vi "check controller rectangle cases.vi"() -> ()   [LabVIEW 2017]
uses:
  <vilib>/Simulation/Scripting/Companion Diagram/SimConfigNode/SimParams.ctl
  <vilib>/Simulation/Scripting/Companion Diagram/SimConfigNode/_simSolvers.ctl
  <vilib>/Simulation/Implementation/Shared/SIMSCR Execution Mode.ctl
  <vilib>/Simulation/Param Hierarchy/Typedefs/SIMPH Param Control Actions.ctl
  <vilib>/Simulation/Implementation/Shared/NILVSim_ParamChanged.vi
  <vilib>/Simulation/Implementation/Shared/NILVSIM_BeginStep.vi
  <vilib>/Simulation/Implementation/Shared/NILVSim_Manager.vi
  <vilib>/Utility/error.llb/Clear Errors.vi
  <vilib>/Simulation/Implementation/Shared/NILVSim_FinalizeModel.vi
  <vilib>/DAQmx/read.llb/DAQmx Read (Counter DBL 1Chan 1Samp).vi
  <vilib>/DAQmx/read.llb/DAQmx Read (Digital Bool 1Line 1Point).vi
  917b7e52-755f-4d44-bea8-9e7c9beac24e.vi
  a58f9967-76f1-4ebc-ad3d-26e75a3ca160.vi
  <vilib>/DAQmx/write.llb/DAQmx Write (Analog DBL 1Chan 1Samp).vi
  <vilib>/DAQmx/create/channels.llb/DAQmx Create Channel (AO-Voltage-Basic).vi
  <vilib>/DAQmx/create/channels.llb/DAQmx Create Channel (DI-Digital Input).vi
  <vilib>/DAQmx/create/channels.llb/DAQmx Create Channel (CI-Count Edges).vi
  <vilib>/Simulation/Implementation/Shared/SIM Unbundle Sim Info.vi
  <vilib>/Simulation/Implementation/Shared/NILVSim_Initialize.vi
  <vilib>/Simulation/Utility/Implementation/NILVSim Get Time and IsAcceptedStep.vi
  <vilib>/Simulation/Implementation/Shared/SIMSH Read Queue.vi
  <vilib>/Simulation/Implementation/Shared/NILVSim_GetModelError.vi
  <vilib>/Simulation/Implementation/Shared/SIM Bundle Sim Info.vi
  <vilib>/DAQmx/miscellaneous.llb/DAQmx Fill In Error Info.vi
  <vilib>/Simulation/Implementation/XNodeFramework/SimXNode/SimX.xnode
  <vilib>/Simulation/Model Libraries/PID/SIM PID (Parallel).vi
  <vilib>/Simulation/Model Libraries/PID/SIM PID.vi
  <vilib>/Simulation/Scripting/Companion Diagram/SimConfigNode/SimDog.xnode
  <vilib>/Simulation/Model Libraries/PID/SIM PID (Academic).vi
  <vilib>/Simulation/Implementation/Shared/NI_SIM_Implementation.lvlib
panel:
  out "Boolean 3":bool
  out "temp height":dbl
  out "Boolean 2":bool
  out "reset":bool
  in  "checking re":bool
  in  "checking enums":T1(ring)
  in  "rectangle":bool
  in  "Boolean":bool
  out "prev index":dbl
  out "Point rectangle is drawing":dbl
  out "Rectangle Y":dbl[](array[numeric])
  out "Rectangle X":dbl[](array[numeric])
  in  "stage rectangle":T2(ring)
  out "Step 2I":bool
  out "Step 2G":bool
  out "Step 2E":bool
  out "stay1":dbl
  out "stay":dbl
  out "calculating error x":dbl
  out "calculating error y":dbl
  in  "origin":bool
  out "Previous Y":dbl
  out "Previous X":dbl
  out "Current Y":dbl
  out "Current X":dbl
  out "previous index":dbl
  out "both/reset enter":bool
  out "reset complete":bool
  out "x circle":bool
  out "y circle":bool
  out "Point circle is drawing":dbl
  out "false":bool
  in  "Radius 2":dbl
  out "No of Points":dbl
  out "Passing Y":dbl
  out "Y array":dbl[](array[numeric])
  out "array Y length 2":dbl
  out "Passing X":dbl
  out "X array":dbl[](array[numeric])
  out "array x Length 2":dbl
  in  "stage circle":T2(ring)
  in  "check instruc":bool
  out "x entered":dbl
  out "y enetred":dbl
  out "greater -1 x":bool
  out "less 1 x":bool
  out "direction selected":dbl
  out "at 2f":bool
  out "Step 2J":bool
  out "Step 2H":bool
  out "Shape drawing steps":enum16{"corner", "1st switch", "reverse"}(ring)
  out "Step 2D":bool
  out "c":bool
  in  "height":dbl
  in  "length":dbl
  in  "part":T3(ring)=enum."a"
  in  "Has encoders been reset?":enum16{"don't reset", "reset"}(ring)
  out "x distance currently being travelled":dbl
  out "y distance currently being travelled":dbl
  out "error calced":dbl
  out "p1 dis 2":dbl
  out "p1 dis":dbl
  out "error y":dbl
  out "calc distance y":dbl
  out "calc distanc x":dbl
  out "error x":dbl
  out "reached y":bool
  out "reached x":bool
  out "Numeric":dbl
  in  "Draw rectangle":bool
  in  "Draw circle":bool
  out "In drawing mode":bool
  in  "Right-Down":bool
  in  "Left-Up":bool
  in  "Left-Down":bool
  in  "Right-Up":bool
  in  "right":bool
  in  "left":bool
  in  "motor 2":dbl(slide)=1.5 scale=-10.0..10.0
  in  "down":bool
  in  "up":bool
  in  "Y Length":dbl=30.0
  in  "X Length":dbl=30.0
  in  "Motor 2 encoder":tag="Dev1/ctr1"
  out "Pulses M2":dbl format="%.2f"
  in  "Motor 1 encoder":tag="Dev1/ctr0"
  out "Pulses M1":dbl format="%.2f"
  out "Right":bool
  out "Bottom":bool
  out "Left":bool
  out "Top":bool
  in  "Switch 4/Line 3":tag="Dev1/port0/line3"
  in  "Switch 3/Line 2":tag="Dev1/port0/line2"
  in  "Switch 2/Line 1":tag="Dev1/port0/line1"
  in  "Switch 1/Line 0":tag="Dev1/port0/line0"
  in  "Motor stop":bool
  in  "Motor 1":tag="Dev1/ao0"
  in  "max Voltage":dbl=10.0
  in  "Min Voltage":dbl=-10.0
  in  "Motor 2":tag="Dev1/ao1"
  in  "motor 1":dbl(slide)=1.5 scale=-10.0..10.0
  in  "stop":bool
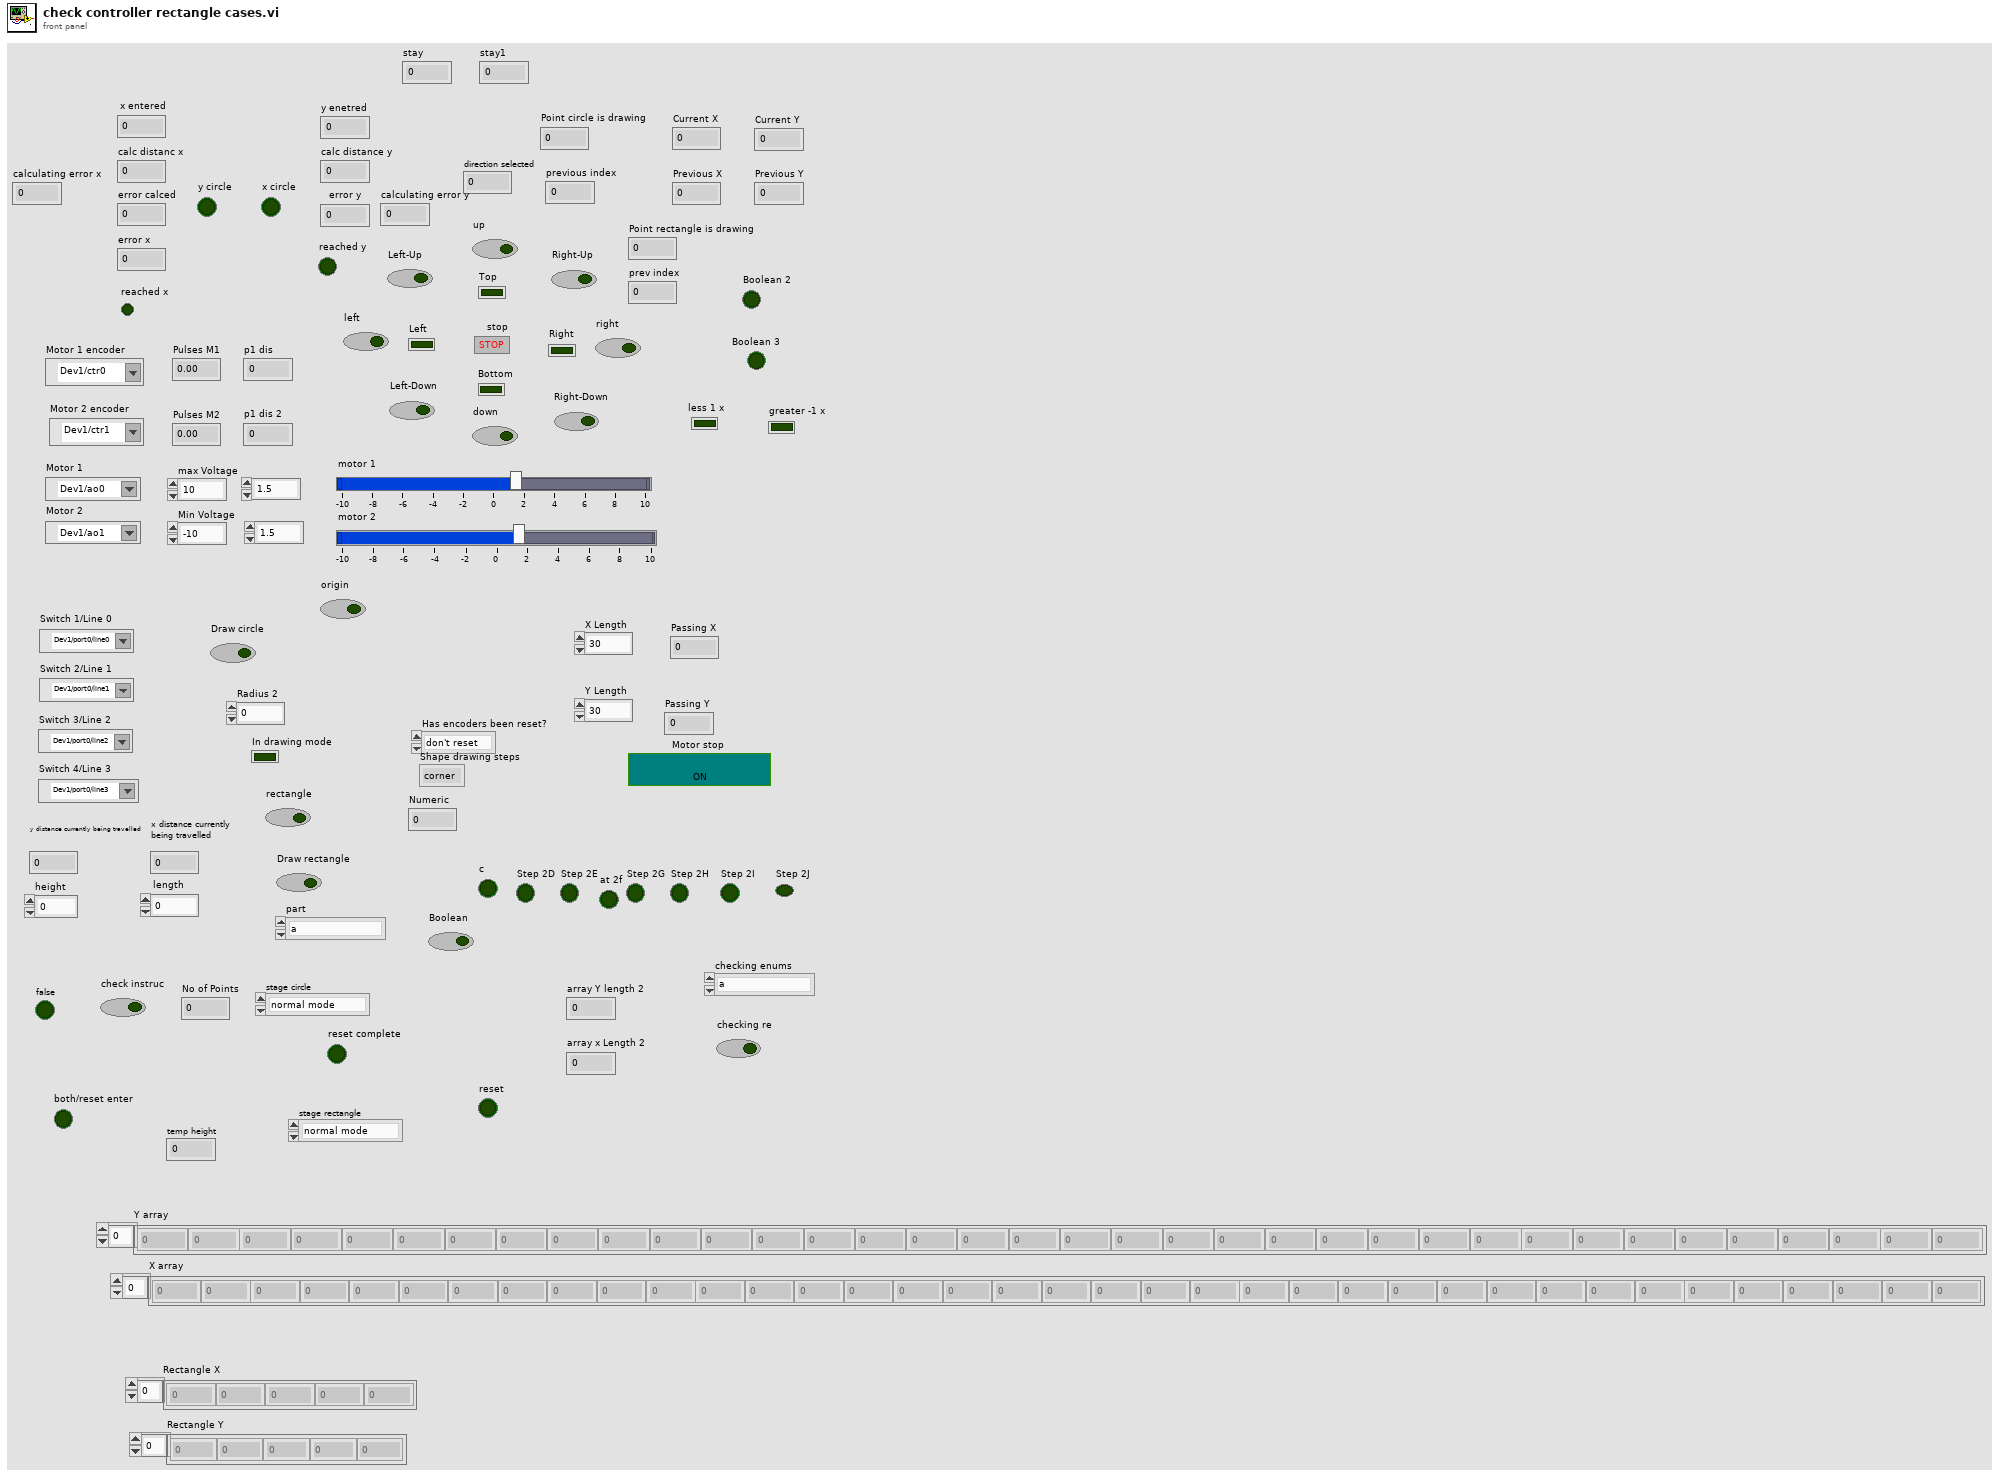
[diagram p1: front panel]
types:
  T1 = enum16{"a", "starting pt", "reset", "going right", "reset before down", "going down", "reset before left", "going left", "reset before up", "going up", "nothing"}
  T2 = enum16{"normal mode", "take to origin", "reset before start", "create points", "draw points", "checking if draw", "reset draw counter"}
  T3 = enum16{"nothing", "j", "i", "h", "g", "f", "e", "d", "c", "b", "a"}
  T4 = enum16{"a", "starting pt", "reset", "going right", "reset before down", "going down", "reset before left", "going left", "reset before up", "going up"}
  T5 = enum16{"Simulate to Completion", "Single Time-Step Simulation (Fixed Step Only)"}
  T6 = typedef "SIMSCR Execution Mode.ctl" = enum16{"Simulate to Completion", "Single Time-Step Simulation (Fixed Step Only)"}
  T7 = typedef "SIMPH Param Control Actions.ctl" = enum16{"get params", "set params"}
  T8 = cluster{"SIMSH Sim Time":dbl, "SIM PID Derivative Gain.vi":cluster{"output":dbl}, "SIM PID Derivative Gain.vi - SIMSH":cluster{"SIMSH Sim Time":dbl, "t 3":dbl, "Select 2":cluster{"s? t:f":dbl}, "Equal?":cluster{"x = y?":bool}, "Or":cluster{"x .or. y?":bool}, "Equal To 0?":cluster{"x = 0?":bool}}, "High Frequency [s] (Tf)":dbl, "Gain":cluster{"output":dbl}, "Summation":cluster{"Result":dbl}, "Integral Gain - series.vi":cluster{"output":dbl}, "Integral Gain - series.vi - SIMSH":cluster{"SIMSH Sim Time":dbl, "Select 2":cluster{"s? t:f":dbl}, "integral in gain?":bool, "Integrator":cluster{"output y(t)":dbl}, "Gain 2":cluster{"output":dbl}, "Select":cluster{"s? t:f":dbl}, "Equal To 0?":cluster{"x = 0?":bool}, "Reciprocal":cluster{"1/x":dbl}}}
  T9 = typedef "SimParams.ctl" = cluster{"Initial Time (s)":dbl, "Final Time (s)":dbl, "Step Size (s)":dbl, "ODE Solver":T10, "Minimum Step Size (s)":dbl, "Maximum Step Size (s)":dbl, "Relative Tolerance":dbl, "Absolute Tolerance":dbl, "Software Timing":bool, "Initial Step Size (s)":dbl, "Automatic Fixed Step Size?":bool, "Automatic Discrete Step Size?":bool, "Discrete Step Size (s)":dbl, "Calculate using Time Step":bool, "Solver Wired?":bool, "Prev.Frm.Expected End":u64, "Prev.Frm.Actual End":u64, "Prev.Frm.Finished Late?":bool, "Prev.Iter.Expected End":u64, "Prev.Iter.Actual End":u64, "Prev.Iter.Finished Late?":bool, "Expected Iteration Start":u64, "Actual Iteration Start":u64, "Expected Frame Start":u64, "Actual Frame Start":u64, "Source Name":string, "Name":string, "Period":i64, "Deadline":i64, "Offset":i64, "Start":i64, "Priority":i32, "Timeout":i32, "Processor":i32, "Mode":enum32{"No Change", "Process missed periods, maintain original phase", "Discard missed periods, maintain original phase", "Process missed periods, ignore original phase", "Discard missed periods, ignore original phase"}, "Wakeup reason":enum32{"Normal", "Aborted", "Asynchronous wakeup", "Timing source error", "Timed loop error", "Timeout"}, "Error":errorcluster, "Source Type":string, "Secondary Source Type":string, "Global End Time":u64, "Global Start Time":u64, "Full Solver Reset":bool, "Execution Mode":T6, "Nan/Inf Check":bool, "Custom Solver Library":string, "Solver Is Variable":bool, "custom solver name":string, "Signal Collection Decimation":u32}
  T10 = typedef "_simSolvers.ctl" = enum16{"Runge-Kutta 1 (Euler)", "Runge-Kutta 2", "Runge-Kutta 3", "Runge-Kutta 4", "Runge-Kutta 23 (variable)", "Runge-Kutta 45 (variable)", "BDF (variable)", "Adams-Moulton (variable)", "Rosenbrock (variable)", "Discrete States Only", "SDIRK 4 (variable)", "Radau 5 (variable)", "Radau 9 (variable)", "Radau 13 (variable)", "Radau [Variable Order] (variable)", "Gear's Method (variable)", "Linearizer", "State Query", "Trim Eval", "Custom Solver"}
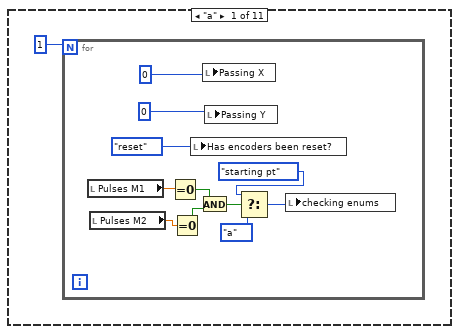
[diagram p3: hidden frame]
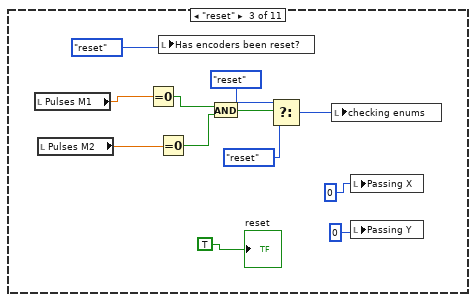
[diagram p4: hidden frame]
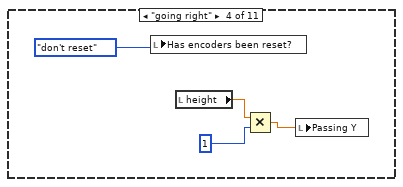
[diagram p5: hidden frame]
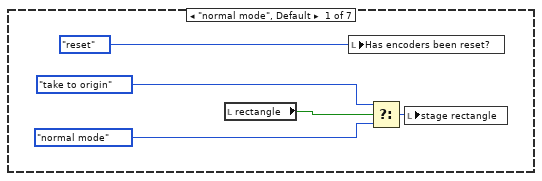
[diagram p14: hidden frame]
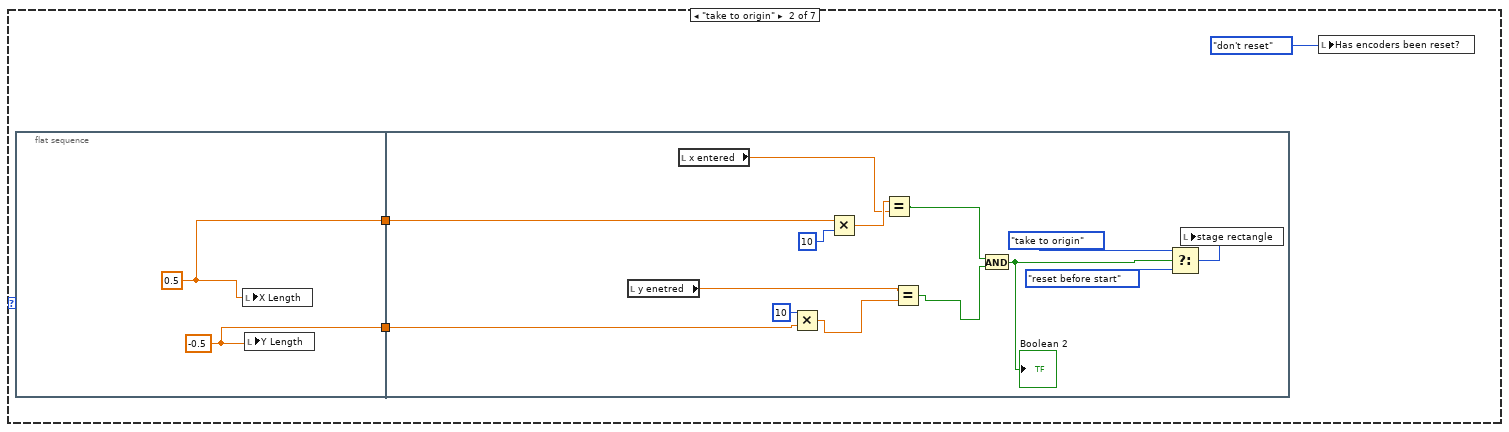
[diagram p15: hidden frame]
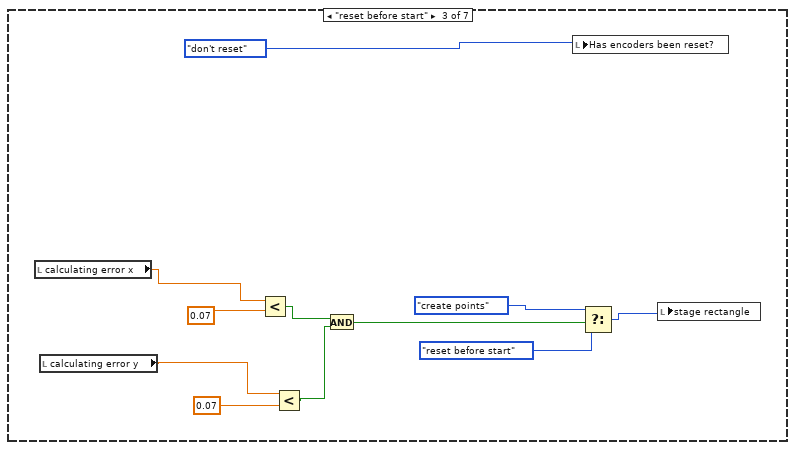
[diagram p16: hidden frame]
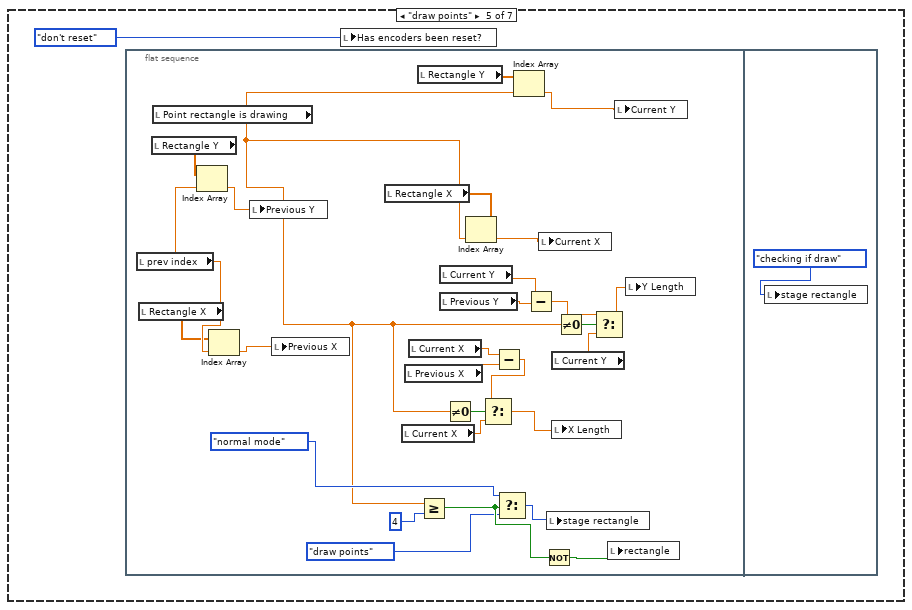
[diagram p17: hidden frame]
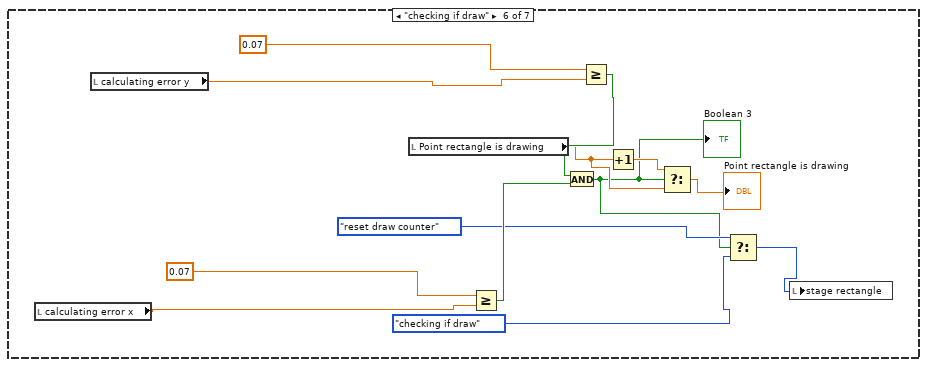
[diagram p18: hidden frame]
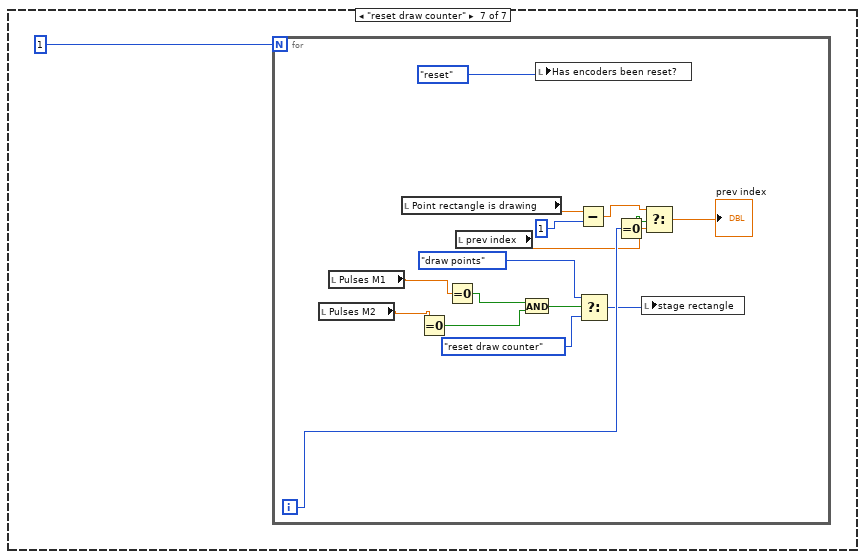
[diagram p19: hidden frame]
diagram:
  n1 = call-poly <vilib>:"DAQmx Create Virtual Channel.vi"("lines"="Switch 1/Line 0") -> ("task out"=w36:refnum<k21>, "error out"=w32:errorcluster)  [unwired: 13 in]
  n2 = call-poly <vilib>:"DAQmx Create Virtual Channel.vi"("lines"="Switch 2/Line 1") -> ("task out"=w35:refnum<k21>, "error out"=w31:errorcluster)  [unwired: 13 in]
  n3 = call-poly <vilib>:"DAQmx Create Virtual Channel.vi"("lines"="Switch 3/Line 2") -> ("task out"=w34:refnum<k21>, "error out"=w30:errorcluster)  [unwired: 13 in]
  n4 = call-poly <vilib>:"DAQmx Create Virtual Channel.vi"("lines"="Switch 4/Line 3") -> ("task out"=w33:refnum<k21>, "error out"=w29:errorcluster)  [unwired: 13 in]
  n5 = call-poly <vilib>:"DAQmx Create Virtual Channel.vi"("maximum value"="max Voltage", "minimum value"="Min Voltage", "physical channels"="Motor 1") -> ("task out"=w46:refnum<k21>, "error out"=w42:errorcluster)  [unwired: 11 in]
  n6 = call <vilib>:"DAQmx Start Task.vi"("task/channels in"=w36, "error in"=w32) -> ("task out"=w28:refnum<k21>, "error out"=w26:errorcluster)  [unwired: 12 in]
  n7 = call <vilib>:"DAQmx Start Task.vi"("task/channels in"=w35, "error in"=w31) -> ("task out"=w24:refnum<k21>, "error out"=w21:errorcluster)  [unwired: 12 in]
  n8 = call-poly <vilib>:"DAQmx Create Virtual Channel.vi"("maximum value"="max Voltage", "minimum value"="Min Voltage", "physical channels"="Motor 2") -> ("task out"=w49:refnum<k21>, "error out"=w41:errorcluster)  [unwired: 11 in]
  n9 = call-poly <vilib>:"DAQmx Create Virtual Channel.vi"("counter"="Motor 1 encoder") -> ("task out"=w7:refnum<k21>, "error out"=w2:errorcluster)  [unwired: 13 in]
  n10 = call-poly <vilib>:"DAQmx Create Virtual Channel.vi"("counter"="Motor 2 encoder") -> ("task out"=w6:refnum<k21>)  [unwired: 13 in, 1 out]
  n11 = call <vilib>:"DAQmx Start Task.vi"("task/channels in"=w34, "error in"=w30) -> ("task out"=w23:refnum<k21>, "error out"=w20:errorcluster)  [unwired: 12 in]
  n12 = call <vilib>:"DAQmx Start Task.vi"("task/channels in"=w33, "error in"=w29) -> ("task out"=w22:refnum<k21>, "error out"=w19:errorcluster)  [unwired: 12 in]
  n13 = call <vilib>:"DAQmx Start Task.vi"("task/channels in"=w7) -> ("task out"=w3:refnum<k21>)  [unwired: 13 in, 1 out]
  n14 = call <vilib>:"DAQmx Start Task.vi"("task/channels in"=w6) -> ("task out"=w1:refnum<k21>)  [unwired: 13 in, 1 out]
  n15 = while {
    tunnel: w49 -> [w242]
    tunnel: [w239] -> w48
    tunnel: w46 -> [w236]
    tunnel: [w235] -> w45
    tunnel: w42 -> [w233]
    tunnel: w41 -> [w232]
    tunnel: w28 -> [w226]
    tunnel: [w225] -> w27
    tunnel: w26 -> [w224]
    tunnel: [w223] -> w25
    tunnel: w24 -> [w222]
    tunnel: w23 -> [w221]
    tunnel: w22 -> [w220]
    tunnel: w21 -> [w219]
    tunnel: w20 -> [w218]
    tunnel: w19 -> [w217]
    tunnel: [w216] -> w18
    tunnel: [w215] -> w17
    tunnel: [w214] -> w16
    tunnel: [w213] -> w15
    tunnel: [w212] -> w14
    tunnel: [w211] -> w13
    tunnel: [w147] -> w10
    tunnel: w3 -> [w149]
    tunnel: w2 -> [w148]
    tunnel: w1 -> [w145]
    stop <- "stop" stop-if-true
    n16 = case shown="True" "check instruc" {
      frame False {
        "false" <- TRUE
      }
      frame True {
        n17 = case shown="\"checking if draw\"" "stage circle" {
          frame "normal mode", Default {
            n18 = local read "check instruc"() -> (w562:bool)
            n19 = local write "Y Length"(0) -> ()
            n20 = local write "X Length"(0) -> ()
            n21 = local write "Has encoders been reset?"(enum16{"don't reset", "reset"}."reset") -> ()
            n22 = Select(t=T2."create points", s=w562, f=T2."normal mode") -> (s? t:f=w563:T2)
            n23 = local write "stage circle"(w563) -> ()
          }
          frame "take to origin" {
            n24 = local write "stage circle"(T2."reset before start") -> ()
            n25 = local write "Has encoders been reset?"(enum16{"don't reset", "reset"}."don't reset") -> ()
          }
          frame "reset before start" {
            n26 = local read "Pulses M1"() -> (w577:dbl)
            n27 = local read "Pulses M2"() -> (w575:dbl)
            n28 = Equal?(x=w577, y=0) -> (x = y?=w572:bool)
            n29 = Equal?(x=w575, y=0) -> (x = y?=w573:bool)
            n30 = local write "Y Length"(0) -> ()
            n31 = local write "X Length"(0) -> ()
            n32 = And(x=w572, y=w573) -> (x .and. y?=w571:bool)
            n33 = local write "Has encoders been reset?"(enum16{"don't reset", "reset"}."reset") -> ()
            n34 = Select(t=T2."create points", s=w571, f=T2."reset before start") -> (s? t:f=w568:T2)
            n35 = local write "stage circle"(w568) -> ()
          }
          frame "create points" {
            n36 = for {
              N: 88 -> [_]
              shift-right: [w597] -> w588
              shift-left: _ -> [_]
              tunnel: [w597] -> w593 mode=indexing
              shift-right: [w596] -> w590
              shift-left: _ -> [_]
              tunnel: [w596] -> w592 mode=indexing
              i -> [w598]
              n37 = Multiply(x=2, y=3.141592653589793) -> (x*y=w601:dbl)
              n38 = Increment(x=w598) -> (x+1=w599:i32)
              n39 = Divide(x=w601, y=88) -> (x/y=w603:dbl)
              n40 = Multiply(x=w603, y=w599) -> (x*y=w600:dbl)
              n41 = Cosine(x=w600) -> (cos(x)=w606:dbl)
              n42 = Sine(x=w600) -> (sin(x)=w607:dbl)
              n43 = Multiply(x=w607, y="Radius 2") -> (x*y=w597:dbl)
              n44 = Multiply(x=w606, y="Radius 2") -> (x*y=w596:dbl)
              "No of Points" <- w598
            }
            "Passing Y" <- w588
            "Y array" <- w593
            "Passing X" <- w590
            "X array" <- w592
            n45 = local read "No of Points"() -> (w587:dbl)
            n46 = Equal?(x=w587, y=87) -> (x = y?=w584:bool)
            n47 = local write "Has encoders been reset?"(enum16{"don't reset", "reset"}."don't reset") -> ()
            n48 = Select(t=T2."draw points", s=w584, f=T2."create points") -> (s? t:f=w594:T2)
            n49 = local write "stage circle"(w594) -> ()
            n50 = Array Size(array=w593) -> (size(s)=→"array Y length 2":i32)
            n51 = Array Size(array=w592) -> (size(s)=→"array x Length 2":i32)
          }
          frame "draw points" {
            n52 = flat-sequence {
              frame #0 {
                n53 = local read "Point circle is drawing"() -> (w636:dbl)
                n54 = local read "previous index"() -> (w628:dbl)
                n55 = local read "Y array"() -> (w629:dbl[])
                n56 = local read "X array"() -> (w630:dbl[])
                n57 = Index Array(array=w629, index=w628) -> (element=→"Previous Y":dbl)
                n58 = Index Array(array=w630, index=w628) -> (element=→"Previous X":dbl)
                n59 = local read "X array"() -> (w631:dbl[])
                n60 = local read "Previous X"() -> (w618:dbl)
                n61 = local read "Current X"() -> (w623:dbl)
                n62 = local read "Y array"() -> (w632:dbl[])
                n63 = local read "Current X"() -> (w621:dbl)
                n64 = Greater Or Equal?(x=w636, y=89) -> (x >= y?=w634:bool)
                n65 = Not Equal To 0?(x=w636) -> (x != 0?=w624:bool)
                n66 = local read "Previous Y"() -> (w619:dbl)
                n67 = local read "Current Y"() -> (w620:dbl)
                n68 = Index Array(array=w631, index=w636) -> (element=→"Current X":dbl)
                n69 = Subtract(x=w621, y=w618) -> (x-y=w616:dbl)
                n70 = Select(t=w616, s=w624, f=w623) -> (s? t:f=w613:dbl)
                n71 = Select(t=T2."normal mode", s=w634, f=T2."draw points") -> (s? t:f=w633:T2)
                n72 = Index Array(array=w632, index=w636) -> (element=→"Current Y":dbl)
                n73 = Subtract(x=w620, y=w619) -> (x-y=w615:dbl)
                n74 = local read "Current Y"() -> (w622:dbl)
                n75 = local write "X Length"(w613) -> ()
                n76 = Not(x=w634) -> (.not. x?=w635:bool)
                n77 = local write "stage circle"(w633) -> ()
                n78 = Not Equal To 0?(x=w636) -> (x != 0?=w625:bool)
                n79 = Select(t=w615, s=w625, f=w622) -> (s? t:f=w614:dbl)
                n80 = local write "Y Length"(w614) -> ()
                n81 = local write "check instruc"(w635) -> ()
              }
              frame #1 {
                n82 = local write "stage circle"(T2."checking if draw") -> ()
              }
            }
            n83 = local write "Has encoders been reset?"(enum16{"don't reset", "reset"}."don't reset") -> ()
          }
          frame "checking if draw" {
            n84 = local read "calculating error x"() -> (w641:dbl)
            n85 = local read "calculating error y"() -> (w639:dbl)
            n86 = local read "Point circle is drawing"() -> (w644:dbl)
            n87 = Greater Or Equal?(x=0.07, y=w641) -> (x >= y?=w647:bool)
            "x circle" <- w647
            n88 = Greater Or Equal?(x=0.07, y=w639) -> (x >= y?=w648:bool)
            "y circle" <- w648
            n89 = And(x=w648, y=w647) -> (x .and. y?=w645:bool)
            "both/reset enter" <- w645
            n90 = Increment(x=w644) -> (x+1=w650:dbl)
            n91 = Select(t=w650, s=w645, f=w644) -> (s? t:f=→"Point circle is drawing":dbl)
            n92 = Select(t=T2."reset draw counter", s=w645, f=T2."checking if draw") -> (s? t:f=w646:T2)
            n93 = local write "stage circle"(w646) -> ()
          }
          frame "reset draw counter" {
            n94 = for {
              N: 1 -> [_]
              i -> [w655]
              n95 = local read "Point circle is drawing"() -> (w660:dbl)
              n96 = local read "Pulses M2"() -> (w665:dbl)
              n97 = local read "Pulses M1"() -> (w666:dbl)
              n98 = Equal To 0?(x=w665) -> (x = 0?=w664:bool)
              n99 = Equal To 0?(x=w666) -> (x = 0?=w662:bool)
              n100 = local read "previous index"() -> (w657:dbl)
              n101 = local write "Has encoders been reset?"(enum16{"don't reset", "reset"}."reset") -> ()
              n102 = And(x=w662, y=w664) -> (x .and. y?=w663:bool)
              n103 = Subtract(x=w660, y=1) -> (x-y=w658:dbl)
              n104 = Select(t=T2."draw points", s=w663, f=T2."reset draw counter") -> (s? t:f=w667:T2)
              n105 = Equal To 0?(x=w655) -> (x = 0?=w654:bool)
              n106 = local write "stage circle"(w667) -> ()
              n107 = Select(t=w658, s=w654, f=w657) -> (s? t:f=→"previous index":dbl)
              "reset complete" <- TRUE
            }
          }
        }
      }
    }
    n108 = case shown="True" "rectangle" {
      frame False {
      }
      frame True {
        n109 = case shown="\"create points\"" "stage rectangle" {
          frame "normal mode", Default {
            n110 = local read "rectangle"() -> (w288:bool)
            n111 = local write "Has encoders been reset?"(enum16{"don't reset", "reset"}."reset") -> ()
            n112 = Select(t=T2."take to origin", s=w288, f=T2."normal mode") -> (s? t:f=w286:T2)
            n113 = local write "stage rectangle"(w286) -> ()
          }
          frame "take to origin" {
            n114 = flat-sequence {
              tunnel: [w295] -> w292
              tunnel: [w294] -> w291
              tunnel: w292 -> [w301]
              tunnel: w291 -> [w300]
              frame #0 {
                w295 = -0.5
                w294 = 0.5
                n115 = local write "X Length"(w294) -> ()
                n116 = local write "Y Length"(w295) -> ()
              }
              frame #1 {
                n117 = local read "y enetred"() -> (w304:dbl)
                n118 = local read "x entered"() -> (w298:dbl)
                n119 = Multiply(x=10, y=w301) -> (x*y=w303:dbl)
                n120 = Multiply(x=w300, y=10) -> (x*y=w299:dbl)
                n121 = Equal?(x=w299, y=w298) -> (x = y?=w297:bool)
                n122 = Equal?(x=w304, y=w303) -> (x = y?=w296:bool)
                n123 = And(x=w297, y=w296) -> (x .and. y?=w309:bool)
                "Boolean 2" <- w309
                n124 = Select(t=T2."take to origin", s=w309, f=T2."reset before start") -> (s? t:f=w308:T2)
                n125 = local write "stage rectangle"(w308) -> ()
              }
            }
            n126 = local write "Has encoders been reset?"(enum16{"don't reset", "reset"}."don't reset") -> ()
          }
          frame "reset before start" {
            n127 = local read "calculating error x"() -> (w312:dbl)
            n128 = local read "calculating error y"() -> (w311:dbl)
            n129 = Less?(x=w312, y=0.07) -> (x < y?=w313:bool)
            n130 = Less?(x=w311, y=0.07) -> (x < y?=w315:bool)
            n131 = And(x=w313, y=w315) -> (x .and. y?=w310:bool)
            n132 = local write "Has encoders been reset?"(enum16{"don't reset", "reset"}."don't reset") -> ()
            n133 = Select(t=T2."create points", s=w310, f=T2."reset before start") -> (s? t:f=w317:T2)
            n134 = local write "stage rectangle"(w317) -> ()
          }
          frame "create points" {
            n135 = local write "Has encoders been reset?"(enum16{"don't reset", "reset"}."reset") -> ()
            n136 = flat-sequence {
              frame #0 {
                n137 = for {
                  N: 1 -> [_]
                  n138 = local read "Rectangle X"() -> (w361:dbl[])
                  n139 = local read "temp height"() -> (w323:dbl)
                  n140 = local read "Rectangle X"() -> (w348:dbl[])
                  n141 = local read "Rectangle X"() -> (w342:dbl[])
                  n142 = local read "Rectangle Y"() -> (w345:dbl[])
                  n143 = local read "Rectangle Y"() -> (w351:dbl[])
                  n144 = local read "length"() -> (w356:dbl)
                  n145 = Insert Into Array(array=w348, index=0, new element=0.05) -> (→"Rectangle X":dbl[])
                  n146 = Insert Into Array(array=w345, index=0, new element=0.05) -> (→"Rectangle Y":dbl[])
                  n147 = Insert Into Array(array=w361, index=2, new element=w356) -> (w358:dbl[])
                  n148 = Insert Into Array(array=w351, index=2, new element=w323) -> (w352:dbl[])
                  n149 = Insert Into Array(array=w342, index=4, new element=0.05) -> (w343:dbl[])
                  n150 = local write "Rectangle X"(w358) -> ()
                  n151 = local write "Rectangle Y"(w352) -> ()
                  n152 = local write "Rectangle X"(w343) -> ()
                  n153 = local read "Rectangle X"() -> (w360:dbl[])
                  n154 = local read "temp height"() -> (w324:dbl)
                  n155 = local read "Rectangle Y"() -> (w349:dbl[])
                  n156 = local read "Rectangle X"() -> (w362:dbl[])
                  n157 = local read "Rectangle Y"() -> (w341:dbl[])
                  n158 = local read "Rectangle Y"() -> (w354:dbl[])
                  n159 = local read "length"() -> (w355:dbl)
                  n160 = Insert Into Array(array=w349, index=1, new element=w324) -> (w350:dbl[])
                  n161 = Insert Into Array(array=w360, index=1, new element=0.05) -> (w357:dbl[])
                  n162 = Insert Into Array(array=w341, index=4, new element=0.05) -> (w344:dbl[])
                  n163 = Insert Into Array(array=w354, index=3, new element=0.05) -> (w353:dbl[])
                  n164 = local write "Rectangle Y"(w350) -> ()
                  n165 = Insert Into Array(array=w362, index=3, new element=w355) -> (w359:dbl[])
                  n166 = local write "Rectangle X"(w357) -> ()
                  n167 = local write "Rectangle Y"(w353) -> ()
                  n168 = local write "Rectangle X"(w359) -> ()
                  n169 = local write "Rectangle Y"(w344) -> ()
                }
              }
              frame #1 {
                n170 = local read "Rectangle X"() -> (w378:dbl[])
                n171 = local read "Rectangle Y"() -> (w377:dbl[])
                n172 = local read "height"() -> (w376:dbl)
                n173 = local read "length"() -> (w372:dbl)
                n174 = Index Array(array=w378, index=2) -> (element=w373:dbl)
                n175 = Index Array(array=w377, index=2) -> (element=w374:dbl)
                n176 = Multiply(x=w376, y=-1) -> (x*y=w375:dbl)
                n177 = Equal?(x=w373, y=w372) -> (x = y?=w371:bool)
                n178 = Equal?(x=w374, y=w375) -> (x = y?=w370:bool)
                n179 = And(x=w371, y=w370) -> (x .and. y?=w363:bool)
                n180 = Select(t=T2."draw points", s=w363, f=T2."create points") -> (s? t:f=w369:T2)
                n181 = local write "stage rectangle"(w369) -> ()
              }
            }
          }
          frame "draw points" {
            n182 = flat-sequence {
              frame #0 {
                n183 = local read "prev index"() -> (w388:dbl)
                n184 = local read "Rectangle X"() -> (w386:dbl[])
                n185 = local read "Rectangle Y"() -> (w387:dbl[])
                n186 = local read "Point rectangle is drawing"() -> (w389:dbl)
                n187 = Index Array(array=w387, index=w388) -> (element=w397:dbl)
                n188 = Index Array(array=w386, index=w388) -> (element=w396:dbl)
                n189 = local write "Previous Y"(w397) -> ()
                n190 = local write "Previous X"(w396) -> ()
                n191 = local read "Rectangle X"() -> (w384:dbl[])
                n192 = local read "Current X"() -> (w391:dbl)
                n193 = local read "Previous X"() -> (w395:dbl)
                n194 = local read "Current X"() -> (w392:dbl)
                n195 = local read "Rectangle Y"() -> (w385:dbl[])
                n196 = Greater Or Equal?(x=w389, y=4) -> (x >= y?=w407:bool)
                n197 = local read "Current Y"() -> (w393:dbl)
                n198 = local read "Previous Y"() -> (w394:dbl)
                n199 = Not Equal To 0?(x=w389) -> (x != 0?=w405:bool)
                n200 = Index Array(array=w384, index=w389) -> (element=w399:dbl)
                n201 = Subtract(x=w392, y=w395) -> (x-y=w403:dbl)
                n202 = Select(t=w403, s=w405, f=w391) -> (s? t:f=w381:dbl)
                n203 = Select(t=T2."normal mode", s=w407, f=T2."draw points") -> (s? t:f=w380:T2)
                n204 = Index Array(array=w385, index=w389) -> (element=w398:dbl)
                n205 = Subtract(x=w393, y=w394) -> (x-y=w402:dbl)
                n206 = local write "Current X"(w399) -> ()
                n207 = Not(x=w407) -> (.not. x?=w383:bool)
                n208 = local write "stage rectangle"(w380) -> ()
                n209 = local read "Current Y"() -> (w390:dbl)
                n210 = local write "X Length"(w381) -> ()
                n211 = Not Equal To 0?(x=w389) -> (x != 0?=w406:bool)
                n212 = Select(t=w402, s=w406, f=w390) -> (s? t:f=w382:dbl)
                n213 = local write "rectangle"(w383) -> ()
                n214 = local write "Current Y"(w398) -> ()
                n215 = local write "Y Length"(w382) -> ()
              }
              frame #1 {
                n216 = local write "stage rectangle"(T2."checking if draw") -> ()
              }
            }
            n217 = local write "Has encoders been reset?"(enum16{"don't reset", "reset"}."don't reset") -> ()
          }
          frame "checking if draw" {
            n218 = local read "calculating error x"() -> (w411:dbl)
            n219 = local read "calculating error y"() -> (w410:dbl)
            n220 = local read "Point rectangle is drawing"() -> (w412:dbl)
            n221 = Greater Or Equal?(x=0.07, y=w411) -> (x >= y?=w419:bool)
            n222 = Greater Or Equal?(x=0.07, y=w410) -> (x >= y?=w420:bool)
            n223 = And(x=w420, y=w419) -> (x .and. y?=w409:bool)
            "Boolean 3" <- w409
            n224 = Increment(x=w412) -> (x+1=w421:dbl)
            n225 = Select(t=w421, s=w409, f=w412) -> (s? t:f=→"Point rectangle is drawing":dbl)
            n226 = Select(t=T2."reset draw counter", s=w409, f=T2."checking if draw") -> (s? t:f=w413:T2)
            n227 = local write "stage rectangle"(w413) -> ()
          }
          frame "reset draw counter" {
            n228 = for {
              N: 1 -> [_]
              i -> [w430]
              n229 = local read "Pulses M2"() -> (w428:dbl)
              n230 = local read "Pulses M1"() -> (w427:dbl)
              n231 = local read "Point rectangle is drawing"() -> (w425:dbl)
              n232 = Equal To 0?(x=w428) -> (x = 0?=w434:bool)
              n233 = Equal To 0?(x=w427) -> (x = 0?=w436:bool)
              n234 = local read "prev index"() -> (w429:dbl)
              n235 = And(x=w436, y=w434) -> (x .and. y?=w435:bool)
              n236 = local write "Has encoders been reset?"(enum16{"don't reset", "reset"}."reset") -> ()
              n237 = Subtract(x=w425, y=1) -> (x-y=w437:dbl)
              n238 = Select(t=T2."draw points", s=w435, f=T2."reset draw counter") -> (s? t:f=w426:T2)
              n239 = Equal To 0?(x=w430) -> (x = 0?=w438:bool)
              n240 = local write "stage rectangle"(w426) -> ()
              n241 = Select(t=w437, s=w438, f=w429) -> (s? t:f=→"prev index":dbl)
            }
          }
        }
      }
    }
    n242 = local read "height"() -> (w51:dbl)
    n243 = Negate(x=w51) -> (-x=w52:dbl)
    n244 = local write "temp height"(w52) -> ()
    n245 = case shown="True" "checking re" {
      frame False {
      }
      frame True {
        n246 = case shown="\"starting pt\"" "checking enums" {
          frame "a" {
            n247 = for {
              N: 1 -> [_]
              n248 = local read "Pulses M1"() -> (w252:dbl)
              n249 = local read "Pulses M2"() -> (w251:dbl)
              n250 = Equal To 0?(x=w252) -> (x = 0?=w250:bool)
              n251 = Equal To 0?(x=w251) -> (x = 0?=w245:bool)
              n252 = local write "Has encoders been reset?"(enum16{"don't reset", "reset"}."reset") -> ()
              n253 = And(x=w250, y=w245) -> (x .and. y?=w249:bool)
              n254 = local write "Passing X"(0) -> ()
              n255 = local write "Passing Y"(0) -> ()
              n256 = Select(t=T4."starting pt", s=w249, f=T4."a") -> (s? t:f=w246:T4)
              n257 = local write "checking enums"(w246) -> ()
            }
          }
          frame "starting pt" {
            n258 = flat-sequence {
              frame #0 {
                n259 = local write "Passing Y"(10) -> ()
                n260 = local write "Passing X"(-6) -> ()
              }
            }
            n261 = local read "calculating error x"() -> (w265:dbl)
            n262 = local read "calculating error y"() -> (w263:dbl)
            n263 = local write "Has encoders been reset?"(enum16{"don't reset", "reset"}."don't reset") -> ()
            n264 = Less?(x=w265, y=0.07) -> (x < y?=w260:bool)
            n265 = Less?(x=w263, y=0.07) -> (x < y?=w261:bool)
            n266 = And(x=w260, y=w261) -> (x .and. y?=w259:bool)
            n267 = Select(t=T4."reset", s=w259, f=T4."starting pt") -> (s? t:f=w256:T4)
            n268 = local write "checking enums"(w256) -> ()
          }
          frame "reset" {
            (unwired) 0
            n269 = local read "Pulses M1"() -> (w279:dbl)
            n270 = local read "Pulses M2"() -> (w278:dbl)
            n271 = Equal To 0?(x=w279) -> (x = 0?=w276:bool)
            n272 = Equal To 0?(x=w278) -> (x = 0?=w277:bool)
            n273 = local write "Has encoders been reset?"(enum16{"don't reset", "reset"}."reset") -> ()
            n274 = And(x=w276, y=w277) -> (x .and. y?=w275:bool)
            n275 = Select(t=T4."reset", s=w275, f=T4."reset") -> (s? t:f=w272:T4)
            n276 = local write "checking enums"(w272) -> ()
            n277 = local write "Passing X"(0) -> ()
            n278 = local write "Passing Y"(0) -> ()
            "reset" <- TRUE
          }
          frame "going right" {
            n279 = local write "Has encoders been reset?"(enum16{"don't reset", "reset"}."don't reset") -> ()
            n280 = local read "height"() -> (w282:dbl)
            n281 = Multiply(x=w282, y=1) -> (x*y=w283:dbl)
            n282 = local write "Passing Y"(w283) -> ()
          }
          frame "reset before down" {
          }
          frame "going down" {
          }
          frame "reset before left" {
          }
          frame "going left" {
          }
          frame "reset before up" {
          }
          frame "going up" {
          }
          frame "nothing" {
          }
        }
      }
    }
    n283 = case shown="True" "Boolean" {
      frame False {
      }
      frame True {
        n284 = case shown="\"d\"" "part" {
          frame "a" {
            n285 = for {
              N: 1 -> [_]
              n286 = local read "Pulses M1"() -> (w447:dbl)
              n287 = local read "Pulses M2"() -> (w446:dbl)
              n288 = Equal To 0?(x=w446) -> (x = 0?=w449:bool)
              n289 = Equal To 0?(x=w447) -> (x = 0?=w448:bool)
              n290 = local write "Has encoders been reset?"(enum16{"don't reset", "reset"}."reset") -> ()
              n291 = And(x=w448, y=w449) -> (x .and. y?=w441:bool)
              n292 = local write "Passing X"(0) -> ()
              n293 = local write "Passing Y"(0) -> ()
              n294 = Select(t=T3."b", s=w441, f=T3."a") -> (s? t:f=w444:T3)
              n295 = local write "part"(w444) -> ()
            }
          }
          frame "b" {
            n296 = local read "calculating error x"() -> (w460:dbl)
            n297 = local read "calculating error y"() -> (w457:dbl)
            n298 = Greater?(x=w460, y=0.07) -> (0:w459:bool)
            n299 = Greater?(x=w457, y=0.07) -> (0:w455:bool)
            n300 = local write "Has encoders been reset?"(enum16{"don't reset", "reset"}."don't reset") -> ()
            n301 = local write "Passing Y"(1) -> ()
            n302 = local write "Passing X"(1) -> ()
            n303 = And(x=w459, y=w455) -> (x .and. y?=w462:bool)
            n304 = Select(t=T3."c", s=w462, f=T3."b") -> (s? t:f=w463:T3)
            n305 = local write "part"(w463) -> ()
          }
          frame "c" {
            n306 = for {
              N: 0 -> [_]
              n307 = local read "Pulses M2"() -> (w476:dbl)
              n308 = local read "Pulses M1"() -> (w475:dbl)
              n309 = Equal To 0?(x=w476) -> (x = 0?=w474:bool)
              n310 = Equal To 0?(x=w475) -> (x = 0?=w473:bool)
              n311 = local write "Has encoders been reset?"(enum16{"don't reset", "reset"}."reset") -> ()
              n312 = And(x=w474, y=w473) -> (x .and. y?=w472:bool)
              n313 = Select(t=T3."d", s=w472, f=T3."c") -> (s? t:f=w469:T3)
              n314 = local write "part"(w469) -> ()
            }
            n315 = local write "Passing Y"(0) -> ()
            n316 = local write "Passing X"(0) -> ()
            "c" <- TRUE
          }
          frame "d" {
            n317 = local read "calculating error y"() -> (w479:dbl)
            n318 = Multiply(x="height", y=-1) -> (x*y=w480:dbl)
            n319 = local write "Has encoders been reset?"(enum16{"don't reset", "reset"}."don't reset") -> ()
            n320 = local write "Passing X"(0) -> ()
            n321 = local write "Passing Y"(w480) -> ()
            n322 = Equal To 0?(x=w479) -> (x = 0?=w478:bool)
            "Step 2D" <- w478
            n323 = Select(t=T3."e", s=w478, f=T3."d") -> (s? t:f=w487:T3)
            n324 = local write "part"(w487) -> ()
          }
          frame "e" {
            n325 = for {
              N: 1 -> [_]
              n326 = local read "Pulses M1"() -> (w494:dbl)
              n327 = local read "Pulses M2"() -> (w493:dbl)
              n328 = Equal To 0?(x=w493) -> (x = 0?=w499:bool)
              n329 = Equal To 0?(x=w494) -> (x = 0?=w500:bool)
              n330 = local write "Has encoders been reset?"(enum16{"don't reset", "reset"}."reset") -> ()
              n331 = And(x=w500, y=w499) -> (x .and. y?=w498:bool)
              n332 = Select(t=T3."f", s=w498, f=T3."e") -> (s? t:f=w492:T3)
              n333 = local write "part"(w492) -> ()
              "Step 2E" <- TRUE
            }
            n334 = local write "Passing X"(0) -> ()
            n335 = local write "Passing Y"(0) -> ()
          }
          frame "f" {
            n336 = local read "calculating error x"() -> (w502:dbl)
            n337 = Equal To 0?(x=w502) -> (x = 0?=w501:bool)
            "at 2f" <- w501
            n338 = local write "Passing Y"(0) -> ()
            n339 = local write "Passing X"("length") -> ()
            n340 = local write "Has encoders been reset?"(enum16{"don't reset", "reset"}."don't reset") -> ()
            n341 = Select(t=T3."g", s=w501, f=T3."f") -> (s? t:f=w506:T3)
            n342 = local write "part"(w506) -> ()
          }
          frame "g" {
            n343 = for {
              N: 1 -> [_]
              n344 = local read "Pulses M1"() -> (w514:dbl)
              n345 = local read "Pulses M2"() -> (w513:dbl)
              n346 = Equal To 0?(x=w514) -> (x = 0?=w521:bool)
              n347 = Equal To 0?(x=w513) -> (x = 0?=w520:bool)
              n348 = local write "Has encoders been reset?"(enum16{"don't reset", "reset"}."reset") -> ()
              n349 = And(x=w521, y=w520) -> (x .and. y?=w519:bool)
              n350 = Select(t=T3."h", s=w519, f=T3."g") -> (s? t:f=w516:T3)
              n351 = local write "part"(w516) -> ()
            }
            n352 = local write "Passing X"(0) -> ()
            n353 = local write "Passing Y"(0) -> ()
            "Step 2G" <- TRUE
          }
          frame "h" {
            n354 = local read "height"() -> (w524:dbl)
            n355 = local read "calculating error y"() -> (w522:dbl)
            n356 = local write "Passing X"(0) -> ()
            n357 = local write "Passing Y"(w524) -> ()
            n358 = local write "Has encoders been reset?"(enum16{"don't reset", "reset"}."don't reset") -> ()
            n359 = Equal To 0?(x=w522) -> (x = 0?=w523:bool)
            n360 = Select(t=T3."i", s=w523, f=T3."h") -> (s? t:f=w527:T3)
            n361 = local write "part"(w527) -> ()
            "Step 2H" <- TRUE
          }
          frame "i" {
            n362 = for {
              N: 1 -> [_]
              n363 = local read "Pulses M1"() -> (w537:dbl)
              n364 = local read "Pulses M2"() -> (w536:dbl)
              n365 = Equal To 0?(x=w536) -> (x = 0?=w542:bool)
              n366 = Equal To 0?(x=w537) -> (x = 0?=w543:bool)
              n367 = And(x=w543, y=w542) -> (x .and. y?=w541:bool)
              n368 = local write "Has encoders been reset?"(enum16{"don't reset", "reset"}."reset") -> ()
              n369 = Select(t=T3."j", s=w541, f=T3."i") -> (s? t:f=w535:T3)
              n370 = local write "part"(w535) -> ()
            }
            n371 = local write "Passing Y"(0) -> ()
            n372 = local write "Passing X"(0) -> ()
            "Step 2I" <- TRUE
          }
          frame "j" {
            n373 = local read "calculating error x"() -> (w548:dbl)
            n374 = local read "length"() -> (w545:dbl)
            n375 = Equal To 0?(x=w548) -> (x = 0?=w547:bool)
            n376 = Multiply(x=w545, y=-1) -> (x*y=w544:dbl)
            n377 = local write "Has encoders been reset?"(enum16{"don't reset", "reset"}."don't reset") -> ()
            n378 = local write "Passing Y"(0) -> ()
            n379 = local write "Passing X"(w544) -> ()
            n380 = Select(t=T3."nothing", s=w547, f=T3."j") -> (s? t:f=w551:T3)
            n381 = local write "part"(w551) -> ()
            "Step 2J" <- TRUE
          }
          frame "nothing" {
            n382 = local write "X Length"(0) -> ()
            n383 = local write "Y Length"(0) -> ()
          }
        }
      }
    }
    n384 = local read "y enetred"() -> (w73:dbl)
    n385 = local read "calc distance y"() -> (w72:dbl)
    n386 = local read "calc distanc x"() -> (w71:dbl)
    n387 = local read "x entered"() -> (w70:dbl)
    n388 = local read "stay"() -> (w67:dbl)
    n389 = local read "stay1"() -> (w66:dbl)
    n390 = formula code="if (Ylength==0)\nYerror=0;\n else  \nif(Ylength<0)\nYerror= Ylength+calculating_y_dis;\nelse\nYerror= Ylength-calculating_y_dis;\n\nif (stay==0)\nYerror=0;"("Ylength"=w73, "calculating_y_dis"=w72, "stay"=w67) -> ("Yerror"=→"error y":dbl)
    n391 = formula code="if (desired_xlength==0)\nXerror=0;\nelse\nif(desired_xlength>0)\nXerror=desired_xlength-actual_xLength;\nelse\nXerror=desired_xlength+actual_xLength;\n\nif (stay1==0)\nXerror=0;"("desired_xlength"=w70, "actual_xLength"=w71, "stay1"=w66) -> ("Xerror"=→"error x":dbl)
    n392 = local read "error y"() -> (w119:dbl)
    n393 = local read "error y"() -> (w118:dbl)
    n394 = local read "error x"() -> (w120:dbl)
    n395 = local read "error y"() -> (w134:dbl)
    n396 = local read "error y"() -> (w131:dbl)
    n397 = local read "error x"() -> (w127:dbl)
    n398 = local read "error x"() -> (w126:dbl)
    n399 = local read "error y"() -> (w135:dbl)
    n400 = local read "error x"() -> (w136:dbl)
    n401 = Less Than 0?(x=w119) -> (x < 0?=w117:bool)
    n402 = Less Than 0?(x=w120) -> (x < 0?=w116:bool)
    n403 = Greater Than 0?(x=w118) -> (x > 0?=w115:bool)
    n404 = Less Than 0?(x=w131) -> (x < 0?=w129:bool)
    n405 = Equal To 0?(x=w136) -> (x = 0?=w130:bool)
    n406 = Greater Than 0?(x=w134) -> (x > 0?=w133:bool)
    n407 = local read "error y"() -> (w112:dbl)
    n408 = local read "error x"() -> (w111:dbl)
    n409 = Greater Than 0?(x=w127) -> (x > 0?=w125:bool)
    n410 = Equal To 0?(x=w135) -> (x = 0?=w124:bool)
    n411 = Less Than 0?(x=w126) -> (x < 0?=w123:bool)
    n412 = And(x=w117, y=w116) -> (x .and. y?=w113:bool)
    n413 = And(x=w116, y=w115) -> (x .and. y?=w114:bool)
    n414 = And(x=w133, y=w130) -> (x .and. y?=w132:bool)
    n415 = And(x=w130, y=w129) -> (x .and. y?=w128:bool)
    n416 = local read "error y"() -> (w107:dbl)
    n417 = And(x=w125, y=w124) -> (x .and. y?=w122:bool)
    n418 = And(x=w124, y=w123) -> (x .and. y?=w121:bool)
    n419 = Greater Than 0?(x=w112) -> (x > 0?=w110:bool)
    n420 = Greater Than 0?(x=w111) -> (x > 0?=w108:bool)
    n421 = Less Than 0?(x=w107) -> (x < 0?=w106:bool)
    n422 = And(x=w110, y=w108) -> (x .and. y?=w109:bool)
    n423 = And(x=w108, y=w106) -> (x .and. y?=w105:bool)
    n424 = Select(t=1, s=w132, f=0) -> (s? t:f=w195:i32)
    n425 = Select(t=10, s=w121, f=0) -> (s? t:f=w193:i32)
    n426 = Select(t=2, s=w128, f=0) -> (s? t:f=w194:i32)
    n427 = Select(t=100, s=w109, f=0) -> (s? t:f=w191:i32)
    n428 = Select(t=200, s=w113, f=0) -> (s? t:f=w190:i32)
    n429 = Select(t=20, s=w122, f=0) -> (s? t:f=w192:i32)
    n430 = Select(t=1000, s=w114, f=0) -> (s? t:f=w189:i32)
    n431 = Select(t=2000, s=w105, f=0) -> (s? t:f=w175:i32)
    n432 = Add(x=w195, y=w194) -> (x+y=w188:i32)
    n433 = Add(x=w193, y=w192) -> (x+y=w187:i32)
    n434 = Add(x=w191, y=w190) -> (x+y=w186:i32)
    n435 = Add(x=w189, y=w175) -> (x+y=w174:i32)
    n436 = Add(x=w188, y=w187) -> (x+y=w185:i32)
    n437 = Add(x=w186, y=w174) -> (x+y=w173:i32)
    n438 = call-poly <vilib>:"DAQmx Read.vi"("task/channels in"=w226, "error in"=w224) -> ("task out"=w225:refnum<k21>, "data"=w157:bool, "error out"=w223:errorcluster)  [unwired: 11 in]
    "Top" <- w157
    n439 = call-poly <vilib>:"DAQmx Read.vi"("task/channels in"=w222, "error in"=w219) -> ("task out"=w216:refnum<k21>, "data"=w166:bool, "error out"=w213:errorcluster)  [unwired: 11 in]
    "Bottom" <- w166
    n440 = call-poly <vilib>:"DAQmx Read.vi"("task/channels in"=w221, "error in"=w218) -> ("task out"=w215:refnum<k21>, "data"=w165:bool, "error out"=w212:errorcluster)  [unwired: 11 in]
    "Right" <- w165
    n441 = call-poly <vilib>:"DAQmx Read.vi"("task/channels in"=w220, "error in"=w217) -> ("task out"=w214:refnum<k21>, "data"=w164:bool, "error out"=w211:errorcluster)  [unwired: 11 in]
    "Left" <- w164
    n442 = Add(x=w185, y=w173) -> (x+y=w104:i32)
    "direction selected" <- w104
    n443 = local read "check instruc"() -> (w79:bool)
    n444 = Multiply(x="Y Length", y=10) -> (x*y=w89:dbl)
    "y enetred" <- w89
    n445 = local read "Pulses M1"() -> (w146:dbl)
    n446 = Boolean To (0,1)(Boolean=w79) -> (0, 1=w78:i16)
    n447 = local read "Pulses M2"() -> (w150:dbl)
    n448 = Divide(x=w146, y=52.56) -> (x/y=→"p1 dis":dbl)
    n449 = feedback #1() -> (w86:dbl)  [unwired: 1 in]
    "calc distance y" <- w86
    n450 = formula code="Yerror=  (abs(Ylength)- abs(calculating_y_dis));\nif (Yerror<0.07)\nstay=0;\nif (stay==0)\nYerror=0;"("Ylength"=w89, "calculating_y_dis"=w86, "stay"=1, "circle"=w78) -> ("Yerror"=w138:dbl, "stay"=→"stay":i32)
    n451 = Divide(x=w150, y=52.56) -> (x/y=→"p1 dis 2":dbl)
    n452 = formula code="X=((PulseM1/52.56)+(PulseM2/52.56))/2.0;\nY=((PulseM1/52.56)+(PulseM2/52.56))/2.0;"("PulseM1"=w146, "PulseM2"=w150) -> ("X"=w53:dbl, "Y"=w54:dbl)
    "calc distanc x" <- w53
    n453 = feedback-in #1(w54) -> ()
    n454 = xnode "PID"("Error"=w138) -> ("Output"=w82:dbl)  [unwired: 2 in, 11 out]
    n455 = Multiply(x="X Length", y=10) -> (x*y=w92:dbl)
    "x entered" <- w92
    n456 = formula code="Xerror=(abs(desired_xlength)-abs(actual_xLength));\n\nif (Xerror<0.07)\nstay1 =0;\nif (stay1==0)\nXerror=0;"("actual_xLength"=w53, "desired_xlength"=w92, "stay1"=1) -> ("Xerror"=w137:dbl, "stay1"=→"stay1":i32)
    "error calced" <- w137
    n457 = case shown="2000" w104 {
      tunnel: "motor 1" -> [w1220 w1223 w1226 w1233 w1237 w1241 w1247 w1253 w1259 w1264 w1271]
      tunnel: "motor 2" -> [w1217 w1225 w1228 w1231 w1236 w1239 w1245 w1251 w1257 w1265 w1270]
      tunnel: [w1216 w1225 w1227 w1230 w1236 w1238 w1244 w1250 w1256 w1262 w1269] -> w90
      tunnel: [w1219 w1222 w1226 w1232 w1237 w1240 w1246 w1252 w1258 w1263 w1268] -> w91
      frame 0, Default {
        n458 = Multiply(x=0, y=w1220) -> (x*y=w1219:dbl)
        n459 = Multiply(x=0, y=w1217) -> (x*y=w1216:dbl)
      }
      frame 1 {
        n460 = Multiply(x=-1, y=w1223) -> (x*y=w1222:dbl)
      }
      frame 2 {
        n461 = Multiply(x=-1.003, y=w1228) -> (x*y=w1227:dbl)
      }
      frame 10 {
        n462 = Multiply(x=-1, y=w1233) -> (x*y=w1232:dbl)
        n463 = Multiply(x=-1.1, y=w1231) -> (x*y=w1230:dbl)
      }
      frame 20 {
      }
      frame 100 {
        n464 = Multiply(x=0, y=w1241) -> (x*y=w1240:dbl)
        n465 = Multiply(x=1, y=w1239) -> (x*y=w1238:dbl)
      }
      frame 200 {
        n466 = Multiply(x=0, y=w1247) -> (x*y=w1246:dbl)
        n467 = Multiply(x=-1, y=w1245) -> (x*y=w1244:dbl)
      }
      frame 1000 {
        n468 = Multiply(x=-1, y=w1253) -> (x*y=w1252:dbl)
        n469 = Multiply(x=0, y=w1251) -> (x*y=w1250:dbl)
      }
      frame 2000 {
        n470 = Multiply(x=1, y=w1259) -> (x*y=w1258:dbl)
        n471 = Multiply(x=0, y=w1257) -> (x*y=w1256:dbl)
      }
      frame 4000 {
        n472 = Multiply(x=-1, y=w1264) -> (x*y=w1263:dbl)
        n473 = Multiply(x=0, y=w1265) -> (x*y=w1262:dbl)
      }
      frame 8000 {
        n474 = Multiply(x=-1, y=w1271) -> (x*y=w1268:dbl)
        n475 = Multiply(x=0, y=w1270) -> (x*y=w1269:dbl)
      }
    }
    n476 = Greater?(x=w82, y=-0.07) -> (0:w77:bool)
    n477 = Less?(x=w82, y=0.07) -> (x < y?=w76:bool)
    n478 = local read "Numeric"() -> (w140:dbl)
    n479 = And(x=w77, y=w76) -> (x .and. y?=w99:bool)
    "reached y" <- w99
    n480 = Multiply(x=0, y=w82) -> (x*y=w103:dbl)
    n481 = Select(t=w103, s=w99, f=w82) -> (s? t:f=→"calculating error y":dbl)
    n482 = Or(x=w166, y=w165) -> (x .or. y?=w209:bool)
    n483 = local read "Draw circle"() -> (w144:bool)
    n484 = And(x=w164, y=w157) -> (x .and. y?=w141:bool)
    n485 = local read "rectangle"() -> (w143:bool)
    n486 = Exclusive Or(1:w157, 2:w164) -> (0:w171:bool)
    n487 = Select(t=1, s=w164, f=0) -> (s? t:f=w156:i32)
    n488 = Select(t=2, s=w157, f=w156) -> (s? t:f=w161:i32)
    n489 = local read "check instruc"() -> (w85:bool)
    n490 = local read "Has encoders been reset?"() -> (w87:enum16{"don't reset", "reset"})
    n491 = xnode "PID 2"("Error"=w137) -> ("Output"=w81:dbl)  [unwired: 2 in, 11 out]
    n492 = Or(x=w144, y=w143) -> (x .or. y?=w84:bool)
    n493 = Select(t=1, s=w171, f=w140) -> (s? t:f=w170:dbl)
    n494 = Select(t=2, s=w141, f=w170) -> (s? t:f=w168:dbl)
    n495 = Or(x=w84, y=w85) -> (x .or. y?=w83:bool)
    n496 = Greater?(x=w81, y=-0.07) -> (0:w95:bool)
    "greater -1 x" <- w95
    n497 = Less?(x=w81, y=0.07) -> (x < y?=w96:bool)
    "less 1 x" <- w96
    n498 = call "Number To Enum.vim"("number"=w161, "enum type"=enum16{"Nothing", "Left", "Top"}."Nothing") -> ("number as enum"=w158:enum16{"Nothing", "Left", "Top"})
    n499 = case shown="True" "origin" {
      selector: "origin" -> [w1193 w1201]
      tunnel: [w1193 w1201] -> w172
      tunnel: w158 -> [_ w1194]
      frame False {
      }
      frame True {
        n500 = local read "Numeric"() -> (w1199:dbl)
        n501 = local read "Shape drawing steps"() -> (w1196:enum16{"corner", "1st switch", "reverse"})
        n502 = Equal?(x=w1199, y=2) -> (x = y?=w1198:bool)
        n503 = Select(t=enum16{"corner", "1st switch", "reverse"}."reverse", s=w1198, f=w1196) -> (s? t:f=w1195:enum16{"corner", "1st switch", "reverse"})
        n504 = case shown="\"reverse\"" w1195 {
          tunnel: w1194 -> [_ w1205 _]
          frame "corner" {
            n505 = local write "Y Length"(50) -> ()
            n506 = local write "Has encoders been reset?"(enum16{"don't reset", "reset"}."don't reset") -> ()
            n507 = local write "X Length"(-50) -> ()
          }
          frame "1st switch" {
            n508 = case shown="\"Nothing\", Default" w1205 {
              frame "Nothing", Default {
                n509 = local write "Y Length"(0) -> ()
                n510 = local write "X Length"(0) -> ()
                n511 = local write "Numeric"(2) -> ()
              }
              frame "Left" {
                n512 = local write "X Length"(0) -> ()
                n513 = local write "Y Length"(50) -> ()
              }
              frame "Top" {
                n514 = local write "X Length"(-50) -> ()
                n515 = local write "Y Length"(0) -> ()
              }
            }
            n516 = local write "Has encoders been reset?"(enum16{"don't reset", "reset"}."don't reset") -> ()
          }
          frame "reverse" {
            n517 = local write "Has encoders been reset?"(enum16{"don't reset", "reset"}."reset") -> ()
            "Numeric" <- 2
          }
        }
      }
    }
    "In drawing mode" <- w172
    n518 = case shown="True" w83 {
      tunnel: w149 -> [w681 w686]
      tunnel: w148 -> [w682 w685]
      tunnel: [w679 w684] -> w147
      frame False {
        n519 = call-poly <vilib>:"DAQmx Read.vi"("task/channels in"=w681, "error in"=w682) -> ("data"=w680:dbl, "error out"=w679:errorcluster)  [unwired: 11 in, 1 out]
        n520 = local write "Pulses M1"(w680) -> ()
      }
      frame True {
        n521 = case shown="\"don't reset\", Default" "Has encoders been reset?" {
          tunnel: w686 -> [w690 w697]
          tunnel: w685 -> [w689 w696]
          tunnel: [w687 w698] -> w684
          frame "don't reset", Default {
            n522 = call-poly <vilib>:"DAQmx Read.vi"("task/channels in"=w690, "error in"=w689) -> ("data"=→"Pulses M1":dbl, "error out"=w687:errorcluster)  [unwired: 11 in, 1 out]
          }
          frame "reset" {
            n523 = call <vilib>:"DAQmx Stop Task.vi"("task/channels in"=w697, "error in"=w696) -> ("task out"=w695:refnum<k21>, "error out"=w694:errorcluster)  [unwired: 12 in]
            n524 = call <vilib>:"DAQmx Start Task.vi"("task/channels in"=w695, "error in"=w694) -> ("task out"=w693:refnum<k21>, "error out"=w692:errorcluster)  [unwired: 12 in]
            n525 = call-poly <vilib>:"DAQmx Read.vi"("task/channels in"=w693, "error in"=w692) -> ("data"=w691:dbl, "error out"=w698:errorcluster)  [unwired: 11 in, 1 out]
            n526 = local write "Pulses M1"(w691) -> ()
          }
        }
      }
    }
    n527 = case shown="True" w83 {
      tunnel: w145 -> [w670 w672]
      tunnel: w87 -> [_ w671]
      frame False {
        n528 = call-poly <vilib>:"DAQmx Read.vi"("task/channels in"=w670) -> ("data"=w669:dbl)  [unwired: 12 in, 2 out]
        n529 = local write "Pulses M2"(w669) -> ()
      }
      frame True {
        n530 = case shown="\"don't reset\", Default" w671 {
          tunnel: w672 -> [w674 w677]
          frame "don't reset", Default {
            n531 = call-poly <vilib>:"DAQmx Read.vi"("task/channels in"=w674) -> ("data"=→"Pulses M2":dbl)  [unwired: 12 in, 2 out]
          }
          frame "reset" {
            n532 = call <vilib>:"DAQmx Stop Task.vi"("task/channels in"=w677) -> ("task out"=w676:refnum<k21>)  [unwired: 13 in, 1 out]
            n533 = call <vilib>:"DAQmx Start Task.vi"("task/channels in"=w676) -> ("task out"=w678:refnum<k21>)  [unwired: 13 in, 1 out]
            n534 = call-poly <vilib>:"DAQmx Read.vi"("task/channels in"=w678) -> ("data"=w675:dbl)  [unwired: 12 in, 2 out]
            n535 = local write "Pulses M2"(w675) -> ()
          }
        }
      }
    }
    n536 = call "Number To Enum.vim"("number"=w168, "enum type"=enum16{"corner", "1st switch", "reverse"}."corner") -> ("number as enum"=→"Shape drawing steps":enum16{"corner", "1st switch", "reverse"})
    n537 = And(x=w95, y=w96) -> (x .and. y?=w98:bool)
    n538 = Multiply(x=0, y=w81) -> (x*y=w101:dbl)
    n539 = feedback-in #2(w98) -> ()
    n540 = feedback #2() -> (w97:bool)  [unwired: 1 in]
    "reached x" <- w97
    n541 = And(x=w99, y=w97) -> (x .and. y?=w155:bool)
    n542 = Or(x=w209, y=w155) -> (x .or. y?=w208:bool)
    n543 = Or(x=w208, y="Motor stop") -> (x .or. y?=w210:bool)
    n544 = Or(x=w210, y="stop") -> (x .or. y?=w230:bool)
    n545 = Select(t=0.0, s=w230, f=w90) -> (s? t:f=w227:dbl)
    n546 = call-poly <vilib>:"DAQmx Write.vi"("task/channels in"=w236, "data"=w227, "error in"=w233) -> ("task out"=w237:refnum<k21>, "error out"=w238:errorcluster)  [unwired: 10 in, 1 out]
    n547 = Select(t=0.0 ("s? t:f"), s=w230, f=w91) -> (s? t:f=w228:dbl)
    n548 = call-poly <vilib>:"DAQmx Write.vi"("task/channels in"=w242, "data"=w228, "error in"=w232) -> ("task out"=w241:refnum<k21>, "error out"=w240:errorcluster)  [unwired: 10 in, 1 out]
    n549 = call <vilib>:"DAQmx Wait Until Done.vi"("task/channels in"=w241, "error in"=w240) -> ("error out"=w239:errorcluster)  [unwired: 12 in, 1 out]
    n550 = call <vilib>:"DAQmx Wait Until Done.vi"("task/channels in"=w237, "error in"=w238) -> ("error out"=w235:errorcluster)  [unwired: 12 in, 1 out]
    n551 = Select(t=w101, s=w97, f=w81) -> (s? t:f=→"calculating error x":dbl)
  }
  n552 = invoke on="motor 1" class="Slide (strict)" method="Reinit To Default"() -> ()  [unwired: 3 in, 3 out]
  n553 = invoke on="Numeric" class="DigNum (strict)" method="Reinit To Default"() -> ()  [unwired: 3 in, 3 out]
  n554 = invoke on="No of Points" class="DigNum (strict)" method="Reinit To Default"() -> ()  [unwired: 3 in, 3 out]
  n555 = invoke on="Shape drawing steps" class="Enum (strict)" method="Reinit To Default"() -> ()  [unwired: 3 in, 3 out]
  n556 = invoke on="part" class="Enum (strict)" method="Reinit To Default"() -> ()  [unwired: 3 in, 3 out]
  n557 = invoke on="stage circle" class="Enum (strict)" method="Reinit To Default"() -> ()  [unwired: 3 in, 3 out]
  n558 = invoke on="array Y length 2" class="DigNum (strict)" method="Reinit To Default"() -> ()  [unwired: 3 in, 3 out]
  n559 = invoke on="c" class="Bool (strict)" method="Reinit To Default"() -> ()  [unwired: 3 in, 3 out]
  n560 = invoke on="at 2f" class="Bool (strict)" method="Reinit To Default"() -> ()  [unwired: 3 in, 3 out]
  n561 = invoke on="reached x" class="Bool (strict)" method="Reinit To Default"() -> ()  [unwired: 3 in, 3 out]
  n562 = invoke on="array x Length 2" class="DigNum (strict)" method="Reinit To Default"() -> ()  [unwired: 3 in, 3 out]
  n563 = invoke on="Step 2D" class="Bool (strict)" method="Reinit To Default"() -> ()  [unwired: 3 in, 3 out]
  n564 = invoke on="Step 2H" class="Bool (strict)" method="Reinit To Default"() -> ()  [unwired: 3 in, 3 out]
  n565 = invoke on="Point circle is drawing" class="DigNum (strict)" method="Reinit To Default"() -> ()  [unwired: 3 in, 3 out]
  n566 = invoke on="reached y" class="Bool (strict)" method="Reinit To Default"() -> ()  [unwired: 3 in, 3 out]
  n567 = invoke on="Step 2E" class="Bool (strict)" method="Reinit To Default"() -> ()  [unwired: 3 in, 3 out]
  n568 = invoke on="Step 2J" class="Bool (strict)" method="Reinit To Default"() -> ()  [unwired: 3 in, 3 out]
  n569 = invoke on="previous index" class="DigNum (strict)" method="Reinit To Default"() -> ()  [unwired: 3 in, 3 out]
  n570 = invoke on="stage rectangle" class="Enum (strict)" method="Reinit To Default"() -> ()  [unwired: 3 in, 3 out]
  n571 = invoke on="Rectangle X" class="Arr (strict)" method="Reinit To Default"() -> ()  [unwired: 3 in, 3 out]
  n572 = invoke on="Rectangle Y" class="Arr (strict)" method="Reinit To Default"() -> ()  [unwired: 3 in, 3 out]
  n573 = invoke on="Point rectangle is drawing" class="DigNum (strict)" method="Reinit To Default"() -> ()  [unwired: 3 in, 3 out]
  n574 = invoke on="prev index" class="DigNum (strict)" method="Reinit To Default"() -> ()  [unwired: 3 in, 3 out]
  n575 = call <vilib>:"Simple Error Handler.vi"("error source (\" \")"="you messed up" ("error source (\" \")"), "error in (no error)"=w48) -> ()  [unwired: 3 in, 5 out]
  n576 = call <vilib>:"Simple Error Handler.vi"("error source (\" \")"="you messed up" ("error source (\" \")"), "error in (no error)"=w45) -> ()  [unwired: 3 in, 5 out]
  n577 = call <vilib>:"DAQmx Clear Task.vi"("task in"=w27, "error in"=w25) -> ()  [unwired: 13 in, 1 out]
  n578 = call <vilib>:"DAQmx Clear Task.vi"("task in"=w17, "error in"=w14) -> ()  [unwired: 13 in, 1 out]
  n579 = call <vilib>:"DAQmx Clear Task.vi"("task in"=w18, "error in"=w15) -> ("error out"=w12:errorcluster)  [unwired: 13 in]
  n580 = call <vilib>:"DAQmx Clear Task.vi"("task in"=w16, "error in"=w13) -> ()  [unwired: 13 in, 1 out]
  n581 = call <vilib>:"Simple Error Handler.vi"("error in (no error)"=w12) -> ()  [unwired: 4 in, 5 out]
  n582 = call <vilib>:"Simple Error Handler.vi"("error source (\" \")"="you messed up" ("error source (\" \")"), "error in (no error)"=w10) -> ()  [unwired: 3 in, 5 out]
